vi "Initialize.vi"(7 "thread ID":i32, 8 "error in (no error)":errorcluster, 9 "component name":string, 10 "Plugin Configuration":refnum<class "Plugin Configuration.lvclass">, 11 "UDP Transceiver in":refnum<class "UDP Transceiver.lvclass">) -> (0 "error out":errorcluster, 3 "UDP Transceiver out":refnum<class "UDP Transceiver.lvclass">)   [LabVIEW 2017, in "UDP Transceiver.lvlib" / "UDP Transceiver.lvclass"]
uses:
  UDP Transceiver.lvclass
  DSF Core.lvlibp/Classes/Configuration/Core/Plugin/Plugin Configuration.lvclass
  DSF Core.lvlibp/Classes/Configuration/Core/Thread/Thread Configuration.lvclass
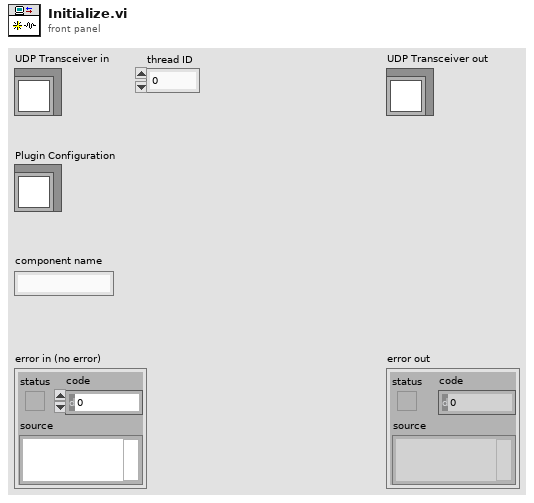
[diagram p1: front panel]
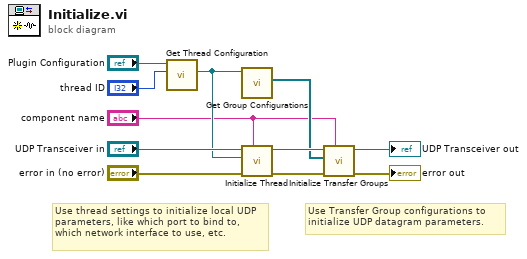
[diagram p0: block diagram]
diagram:
  # "Use thread settings to initialize local UDP parameters, like which port to bind to, which network interface to use, etc."
  # "Use Transfer Group configurations to initialize UDP datagram parameters."
  n1 = call "Get Thread Configuration.vi"("index"="thread ID", "Plugin Configuration in"="Plugin Configuration") -> ("Thread Configuration"=w2:refnum<class "Thread Configuration.lvclass">)  [unwired: 7 in, 2 out]
  n2 = call "Get Group Configurations.vi"("Thread Configuration in"=w2) -> ("Group Configurations"=w3:refnum<class "Group Configuration.lvclass">[])  [unwired: 8 in, 2 out]
  n3 = call-dynamic "Initialize Thread.vi"("component name"="component name", "error in (no error)"="error in (no error)", "Thread Configuration"=w2, "UDP Transceiver in"="UDP Transceiver in") -> ("error out"=w6:errorcluster, "UDP Transceiver out"=w8:refnum<class "UDP Transceiver.lvclass">)  [unwired: 6 in]
  n4 = call-dynamic "Initialize Transfer Groups.vi"("component name"="component name", "error in (no error)"=w6, "Group Configurations"=w3, "UDP Transceiver in"=w8) -> ("error out"=→"error out":errorcluster, "UDP Transceiver out"=→"UDP Transceiver out":refnum<class "UDP Transceiver.lvclass">)  [unwired: 6 in]
